vi "Communcation Bus Dialog.vi"(8 "error in":errorcluster, 11 "Config in":refnum<class "Config.lvclass">) -> (0 "error out":errorcluster, 3 "Config out":refnum<class "Config.lvclass">)   [LabVIEW 2023, in "Config.lvlib" / "Config.lvclass"]
uses:
  Config.lvclass
  Config.lvclass/Config.ctl
panel:
  in  "Prev Resource":string
  in  "Use Previous":bool
  out "Dialog":string
  in  "SEL_NO_Resource":bool
  in  "Str_Resource":string
  in  "SEL_Str_Resource":bool
  in  "Resource":refnum<visa-resource-name>
  in  "SEL_VISA":bool
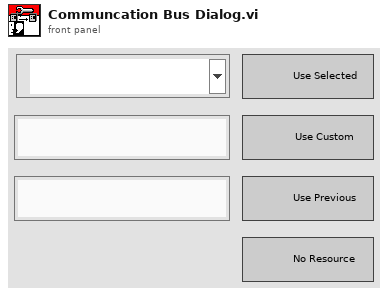
[diagram p1: front panel]
types:
  T1 = enum8{"Enabled", "Disabled", "Disabled and Grayed Out"}
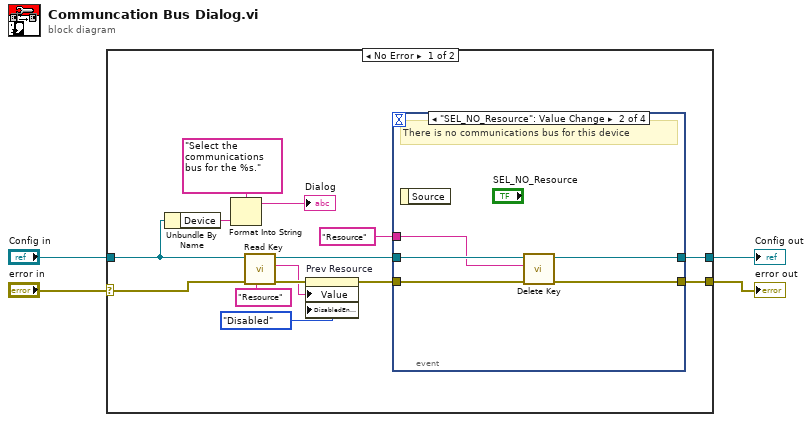
[diagram p0: block diagram]
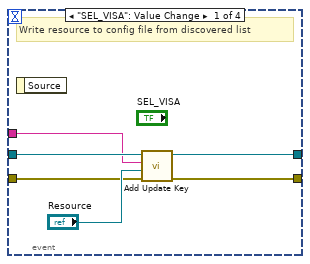
[diagram p2: hidden frame]
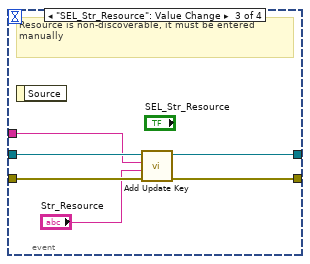
[diagram p3: hidden frame]
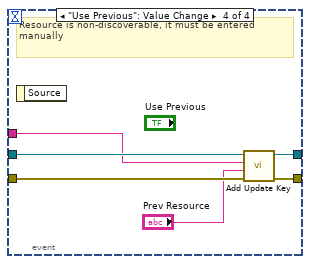
[diagram p4: hidden frame]
diagram:
  n1 = case shown="No Error" "error in" {
    selector: "error in" -> [w5 w42]
    tunnel: [w18 w43] -> w4
    tunnel: [w17 w42] -> w3
    tunnel: "Config in" -> [w12 w43]
    frame No Error {
      n2 = Unbundle By Name(w12) -> ("Device"=w15:string)
      n3 = Format Into String(format string="Select the communications bus for the %s.", w15) -> (resulting string=→"Dialog":string)  [unwired: 2 in, 1 out]
      n4 = call "Read Key.vi"("Key Name"="Resource", "error in"=w5, "Config in"=w12) -> ("error out"=w10:errorcluster, "Key Value"=w8:string, "Config out"=w11:refnum<class "Config.lvclass">)  [unwired: 6 in]
      n5 = property on="Prev Resource" class="Str"(error in=w10, "Value"=w8, "DisabledEnum"=T1."Disabled" ("Disabled")) -> (error out=w9:errorcluster)  [unwired: 1 in, 1 out]
      n6 = event shown="[1] \"SEL_NO_Resource\": Value Change" {
        selector: _ -> [_ _ _ _]
        dyn-events: _ -> [_ _ _ _]
        timeout: _ -> [_ _ _ _]
        tunnel: w11 -> [w24 w29 w35 w41]
        tunnel: [w23 w28 w34 w40] -> w18
        tunnel: [w21 w27 w33 w39] -> w17
        tunnel: w9 -> [w20 w26 w32 w38]
        tunnel: "Resource" -> [w19 w25 w30 w36]
        event "SEL_VISA": Value Change {
          # "Write resource to config file from discovered list"
          n7 = event-data() -> ()  [unwired: 1 in, 1 out]
          n8 = call "Add Update Key.vi"("error in"=w20, "Value"="Resource", "Key"=w19, "Config in"=w24) -> ("error out"=w21:errorcluster, "Config out"=w23:refnum<class "Config.lvclass">)  [unwired: 6 in]
        }
        event "SEL_NO_Resource": Value Change {
          # "There is no communications bus for this device"
          n9 = event-data() -> ()  [unwired: 1 in, 1 out]
          n10 = call "Delete Key.vi"("error in"=w26, "Key"=w25, "Config in"=w29) -> ("error out"=w27:errorcluster, "Config out"=w28:refnum<class "Config.lvclass">)  [unwired: 7 in]
        }
        event "SEL_Str_Resource": Value Change {
          # "Resource is non-discoverable, it must be entered manually"
          n11 = event-data() -> ()  [unwired: 1 in, 1 out]
          n12 = call "Add Update Key.vi"("error in"=w32, "Value"="Str_Resource", "Key"=w30, "Config in"=w35) -> ("error out"=w33:errorcluster, "Config out"=w34:refnum<class "Config.lvclass">)  [unwired: 6 in]
        }
        event "Use Previous": Value Change {
          # "Resource is non-discoverable, it must be entered manually"
          n13 = event-data() -> ()  [unwired: 1 in, 1 out]
          n14 = call "Add Update Key.vi"("error in"=w38, "Value"="Prev Resource", "Key"=w36, "Config in"=w41) -> ("error out"=w39:errorcluster, "Config out"=w40:refnum<class "Config.lvclass">)  [unwired: 6 in]
        }
      }
    }
    frame Error {
    }
  }
  "error out" <- w3
  "Config out" <- w4
